vi "Get Input Script Init.vi"(8 "error in (no error)":errorcluster, 11 "Device Type":u32) -> (0 "error out":errorcluster, 1 "Force Targets":dbl[](array[numeric]), 4 "Variable Dwell":dbl[](array[numeric]), 5 "PID":T1)   [LabVIEW 2013]
uses:
  <vilib>/Utility/NIReport.llb/NI_report.lvclass
  InputScript states.ctl
  <vilib>/Utility/NIReport.llb/Excel/NI_Excel.lvclass
  <vilib>/addons/_office/NI_ReportGenerationToolkit.lvlib
  <vilib>/addons/_office/excel.llb/Excel Get Data ([dbl]).vi
panel:
  in  "State":T2
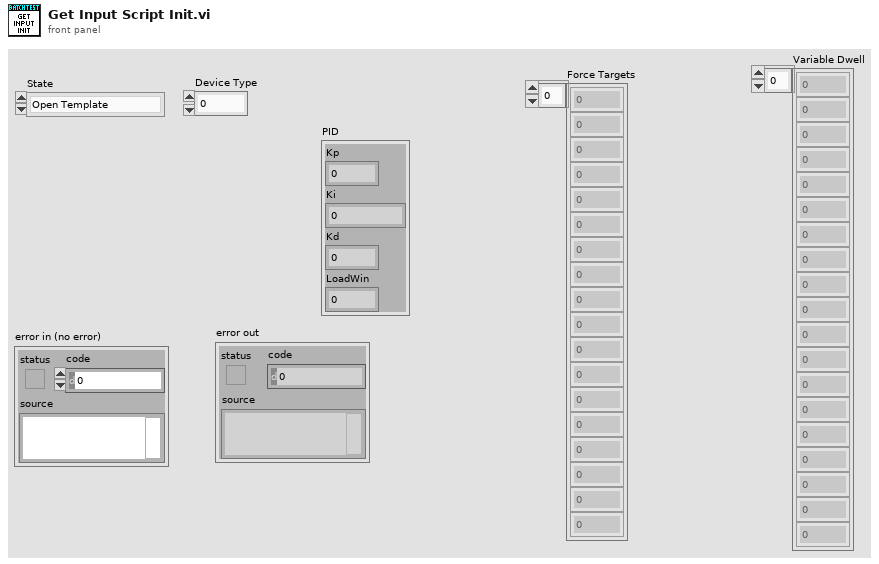
[diagram p1: front panel]
types:
  T1 = cluster{"Kp":dbl, "Ki":dbl, "Kd":dbl, "LoadWin":dbl}
  T2 = typedef "InputScript states.ctl" = enum16{"Open Template", "Write Values", "Read Results", "Close Template"}
  T3 = enum16{"Standard Report", "HTML", "Word", "Excel"}
  T4 = cluster{"data[0]":dbl, "data[1]":dbl, "data[2]":dbl, "data[3]":dbl, "data[4]":dbl, "data[5]":dbl, "data[6]":dbl, "data[7]":dbl, "data[8]":dbl}
  T5 = cluster{"data[0]":dbl, "data[1]":dbl, "data[2]":dbl, "data[3]":dbl}
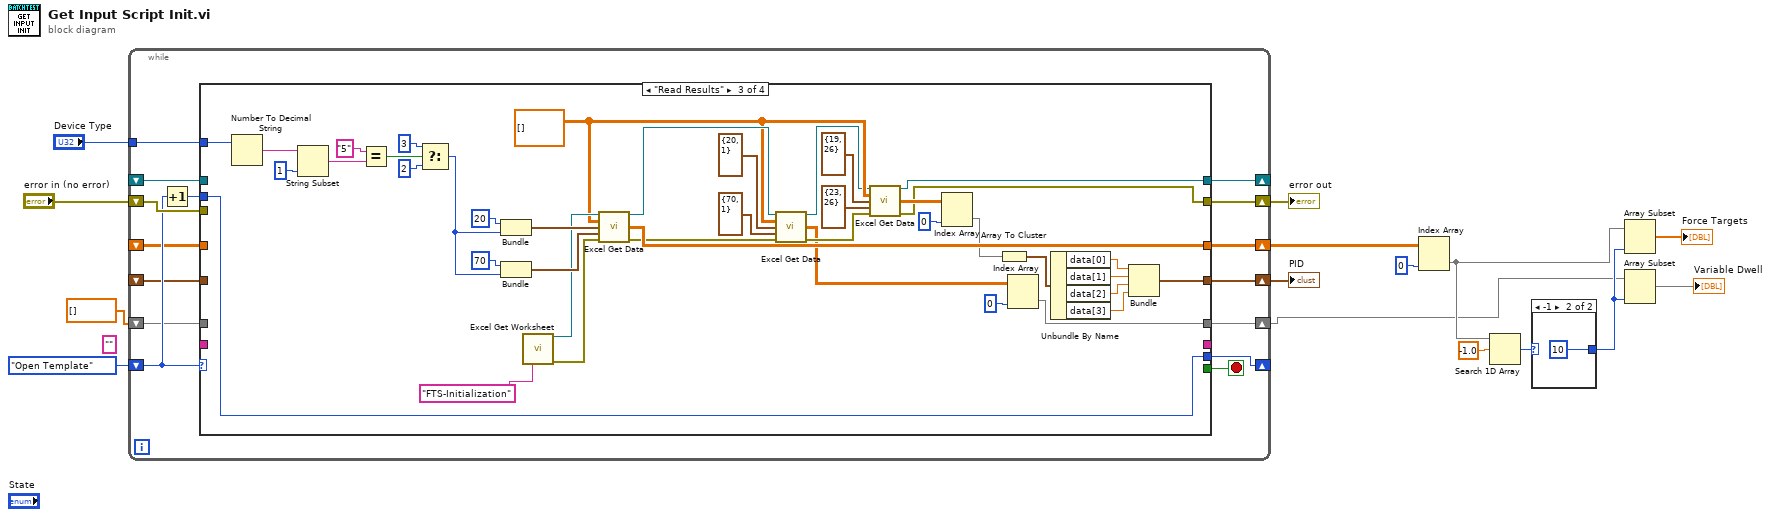
[diagram p0: block diagram]
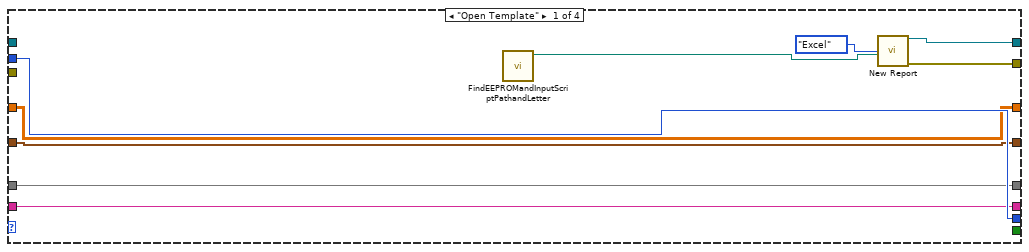
[diagram p3: hidden frame]
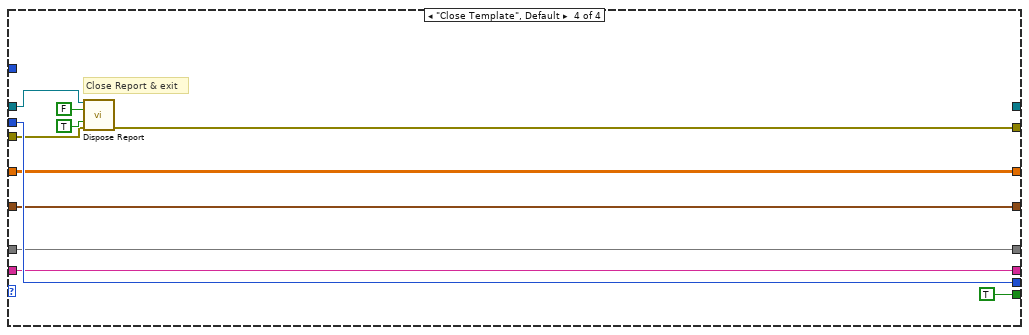
[diagram p5: hidden frame]
diagram:
  (unwired) "" ("Input Script Letter")
  n1 = while {
    shift-right: [w30] -> _
    shift-left: _ -> [w29]
    shift-right: [w28] -> w13
    shift-left: "error in (no error)" -> [w27]
    shift-right: [w24] -> _
    shift-left: InputScript_states."Open Template" -> [w26]
    tunnel: "Device Type" -> [w22]
    shift-right: [w21] -> w6
    shift-left: _ -> [w20]
    shift-right: [w18] -> w5
    shift-left: _ -> [w19]
    shift-right: [w17] -> w2
    shift-left: dbl[] [] ("data") -> [w16]
    stop <- w31 stop-if-true
    n2 = Increment(x=w26) -> (x+1=w25:T2)
    n3 = case shown="\"Read Results\"" w26 {
      tunnel: [_ _ _ TRUE] -> w31
      tunnel: [w40 w47 w48 _] -> w30
      tunnel: w29 -> [_ w47 w87 w91]
      tunnel: [w39 w46 w49 w99] -> w28
      tunnel: w27 -> [_ w46 _ w90]
      tunnel: w25 -> [w38 w45 w89 w97]
      tunnel: [w38 w45 w89 w97] -> w24
      tunnel: [w37 w44 _ w96] -> _
      tunnel: [w37 w44 _ w96] -> w23
      tunnel: w22 -> [_ _ w76 _]
      tunnel: [w36 w43 w71 w95] -> w21
      tunnel: w20 -> [w36 w43 _ w95]
      tunnel: [w35 w41 w72 w94] -> w17
      tunnel: w16 -> [w35 w41 _ w94]
      tunnel: [w34 w42 w77 w93] -> w18
      tunnel: w19 -> [w34 w42 _ w93]
      frame "Open Template" {
        n4 = call "FindEEPROMandInputScriptPathandLetter.vi"() -> ("Template Path"=w32:path)  [unwired: 7 in, 2 out]
        n5 = call <vilib>:"New Report.vi"("report type"=T3."Excel", "template (empty)"=w32) -> ("report out"=w40:refnum<class "NI_report.lvclass">, "error out"=w39:errorcluster)  [unwired: 12 in]
      }
      frame "Write Values" {
      }
      frame "Read Results" {
        w54 = dbl[][] [] ("data type")
        n6 = Number To Decimal String(number=w76) -> (decimal integer string=w75:string)  [unwired: 1 in]
        n7 = String Subset(string=w75, length (rest)=1 ("length (rest)")) -> (substring=w69:string)  [unwired: 1 in]
        n8 = Equal?(x="5", y=w69) -> (x = y?=w70:bool)
        n9 = Select(t=3 ("column"), s=w70, f=2 ("column")) -> (s? t:f=w62:i32)
        n10 = Bundle("row"=20, "column"=w62) -> (w65:cluster{"row":i32, "column":i32})  [unwired: 1 in]
        n11 = Bundle("row"=70, "column"=w62) -> (w61:cluster{"row":i32, "column":i32})  [unwired: 1 in]
        n12 = call <vilib>:"Excel Get Worksheet.vi"("name (\"\")"="FTS-Initialization" ("name (\"\")")) -> ("report out"=w58:refnum<class "NI_report.lvclass">, "error out"=w60:errorcluster)  [unwired: 13 in]
        n13 = call-poly <vilib>:"Excel Get Data.vi"("report in"=w58, "data type"=w54, "start (-1, -1)"=w65, "end (-1, -1)"=w61, "error in (no error)"=w60) -> ("report out"=w55:refnum<class "NI_report.lvclass">, "data"=w71:dbl[][], "error out"=w57:errorcluster)  [unwired: 8 in]
        n14 = call-poly <vilib>:"Excel Get Data.vi"("report in"=w55, "data type"=w54, "start (-1, -1)"=cluster{"row":i32, "column":i32} {"row"=20, "column"=1}, "end (-1, -1)"=cluster{"row":i32, "column":i32} {"row"=70, "column"=1} ("start (-1, -1)"), "error in (no error)"=w57) -> ("report out"=w50:refnum<class "NI_report.lvclass">, "data"=w51:dbl[][], "error out"=w56:errorcluster)  [unwired: 8 in]
        n15 = call-poly <vilib>:"Excel Get Data.vi"("report in"=w50, "data type"=w54, "start (-1, -1)"=cluster{"row":i32, "column":i32} {"row"=19, "column"=26}, "end (-1, -1)"=cluster{"row":i32, "column":i32} {"row"=23, "column"=26}, "error in (no error)"=w56) -> ("report out"=w48:refnum<class "NI_report.lvclass">, "data"=w84:dbl[][], "error out"=w49:errorcluster)  [unwired: 8 in]
        n16 = Index Array(array=w84, index (col)=0 ("index (row)")) -> (element=w59:dbl[])  [unwired: 1 in]
        n17 = Array To Cluster(array=w59) -> (cluster=w82:T4)
        n18 = Index Array(array=w51, index (col)=0 ("index (row)")) -> (element=w72:dbl[])  [unwired: 1 in]
        n19 = Unbundle By Name(w82) -> ("data[0]"=w81:dbl, "data[1]"=w80:dbl, "data[2]"=w79:dbl, "data[3]"=w78:dbl)
        n20 = Bundle("data[0]"=w81, "data[1]"=w80, "data[2]"=w79, "data[3]"=w78) -> (w77:T5)  [unwired: 1 in]
      }
      frame "Close Template", Default {
        # "Close Report & exit"
        n21 = call-dynamic "Dispose Report.vi"("report in"=w91, "wait until printing completed? (T)"=FALSE, "save changes? (F)"=TRUE, "error in (no error)"=w90) -> ("error out"=w99:errorcluster)  [unwired: 11 in]
      }
    }
  }
  "error out" <- w13
  "PID" <- w5
  n22 = Index Array(array=w6, index (col)=0 ("index (row)")) -> (element=w8:dbl[])  [unwired: 1 in]
  n23 = Search 1D Array(1D array=w8, element=-1.0) -> (index of element=w9:i32)  [unwired: 1 in]
  n24 = case shown="-1" w9 {
    selector: w9 -> [w101 _]
    tunnel: [w101 10 ("index of element")] -> w7
    frame Default {
    }
    frame -1 {
    }
  }
  n25 = Array Subset(array=w8, length=w7) -> (→"Force Targets":dbl[])  [unwired: 1 in]
  n26 = Array Subset(array=w2, length=w7) -> (→"Variable Dwell":dbl[])  [unwired: 1 in]
